vi "Channel String to Number of Channels.vi"(4 "Channels String":string="PXI1Slot2/ai1:3") -> (1 "# channels":i32)   [LabVIEW 2016, in "LockinDAQ.lvclass"]
uses:
  LockinDAQ.lvclass
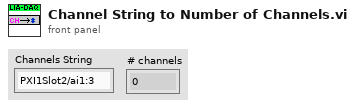
[diagram p1: front panel]
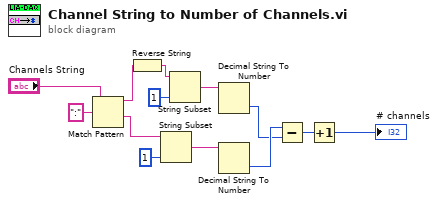
[diagram p0: block diagram]
diagram:
  n1 = Match Pattern(string="Channels String", regular expression=":") -> (before substring=w3:string, after substring=w7:string)  [unwired: 1 in, 2 out]
  n2 = Reverse String(1:w3) -> (0:w2:string)
  n3 = String Subset(string=w7, length (rest)=1 ("length (rest)")) -> (substring=w8:string)  [unwired: 1 in]
  n4 = String Subset(string=w2, length (rest)=1 ("length (rest)")) -> (substring=w9:string)  [unwired: 1 in]
  n5 = Decimal String To Number(string=w9) -> (number=w5:i32)  [unwired: 2 in, 1 out]
  n6 = Decimal String To Number(string=w8) -> (number=w6:i32)  [unwired: 2 in, 1 out]
  n7 = Subtract(x=w6, y=w5) -> (x-y=w4:i32)
  n8 = Increment(x=w4) -> (x+1=→"# channels":i32)
